vi "Set Z Voltage.vi"(2 "Z position (V)":dbl) -> ()   [LabVIEW 2014]
uses:
  global_channels.vi
  global_variables_AWG.vi
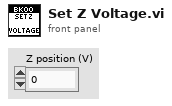
[diagram p1: front panel]
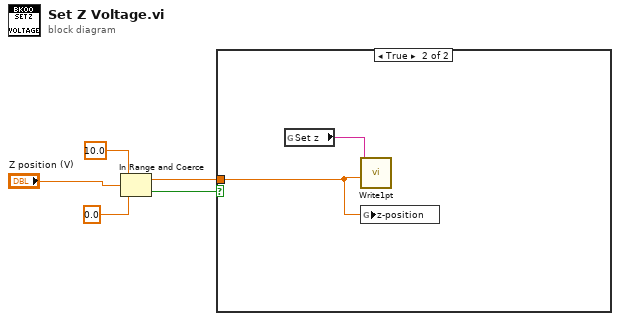
[diagram p0: block diagram]
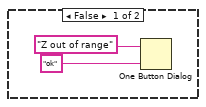
[diagram p2: hidden frame]
diagram:
  n1 = In Range and Coerce(upper limit=10.0, x="Z position (V)", lower limit=0.0) -> (coerced(x)=w1:dbl, In Range?=w2:bool)
  n2 = case shown="True" w2 {
    tunnel: w1 -> [_ w8]
    frame False {
      n3 = One Button Dialog(message="Z out of range", button name ("OK")="ok") -> ()  [unwired: 1 out]
    }
    frame True {
      n4 = global read "global_channels.vi" "Set z"() -> (w9:tag)
      n5 = call "Write1pt.vi"("data"=w8, "physical channel"=w9) -> ()  [unwired: 10 in]
      n6 = global write "global_variables_AWG.vi" "z-position"(w8) -> ()
    }
  }
